vi "table name.vi"(2 "postfix":string, 3 "object name":string) -> (1 "table name":string)   [LabVIEW 2019, in "PostgreSQL.lvlib"]
uses:
  PostgreSQL.lvlib
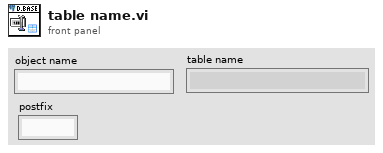
[diagram p1: front panel]
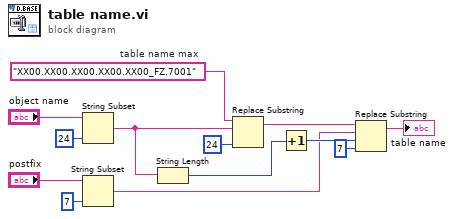
[diagram p0: block diagram]
diagram:
  w12 = "XX00.XX00.XX00.XX00.XX00_FZ.7001"  # table name max
  n1 = String Subset(string="object name", length (rest)=24 ("length (rest)")) -> (substring=w7:string)  [unwired: 1 in]
  n2 = String Subset(string="postfix", length (rest)=7 ("length (rest)")) -> (substring=w1:string)  [unwired: 1 in]
  n3 = String Length(string=w7) -> (length=w11:i32)
  n4 = Replace Substring(2:24 ("length (rest)"), 4:w7, 5:w12) -> (1:w9:string)  [unwired: 1 in, 1 out]
  n5 = Increment(x=w11) -> (x+1=w13:i32)
  n6 = Replace Substring(2:7 ("length (len. of substring)"), 3:w13, 4:w1, 5:w9) -> (1:→"table name":string)  [unwired: 1 out]
